vi "Data 2 TypeDescriptor.vi"(8 "error in (no error)":errorcluster, 11 "Data":variant) -> (0 "Error Out":errorcluster, 3 "TypeDescriptor":string)   [LabVIEW 2014, in "CS++Utilities.lvlib"]
uses:
  CS++Utilities.lvlib
  <vilib>/Utility/VariantDataType/VariantType.lvlib
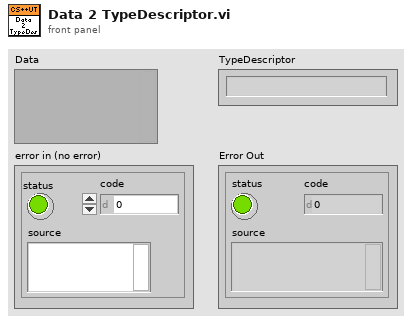
[diagram p1: front panel]
types:
  T1 = typedef "VariantType.lvlib/Type.ctl" = enum8{"Invalid Type", "Void", "I8", "I16", "I32", "I64", "U8", "U16", "U32", "U64", "Single Float", "Double Float", "Extended Float", "Single Complex", "Double Complex", "Extended Complex", "Enum U8", "Enum U16", "Enum U32", "Enum U64", "Single Float With Unit", "Double Float With Unit", "Extended Float With Unit", "Single Complex with Unit", "Double Complex with Unit", "Extended Complex with Unit", "Boolean", "String", "Path", "Picture", "Tag", "Array", "Cluster", "Variant", "LV Variant", "Waveform", "Timestamp", "Digital Waveform", "Digital Data", "ExpressData", "Refnum", "External Data", "VI", "Poly VI", "LabVIEW Class Instance", "Fixed Point"}
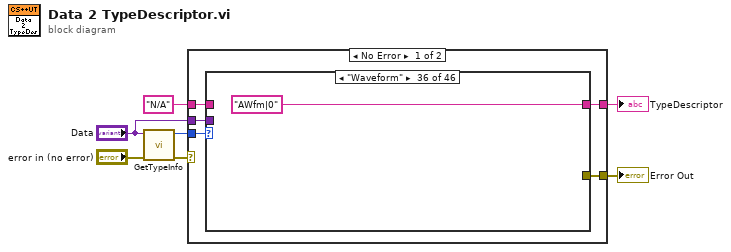
[diagram p0: block diagram]
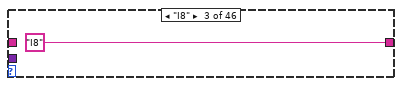
[diagram p4: hidden frame]
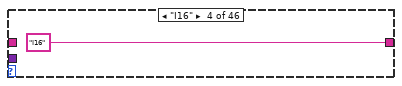
[diagram p5: hidden frame]
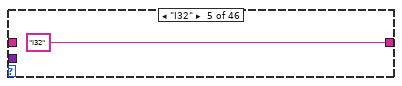
[diagram p6: hidden frame]
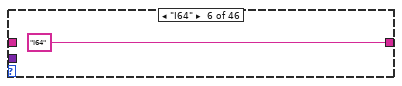
[diagram p7: hidden frame]
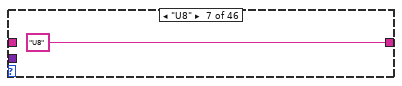
[diagram p8: hidden frame]
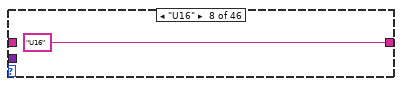
[diagram p9: hidden frame]
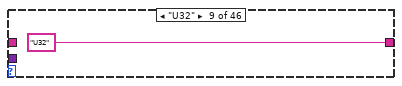
[diagram p10: hidden frame]
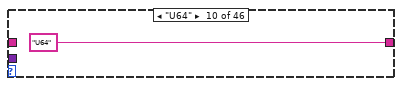
[diagram p11: hidden frame]
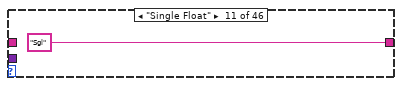
[diagram p12: hidden frame]
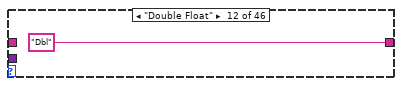
[diagram p13: hidden frame]
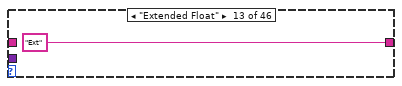
[diagram p14: hidden frame]
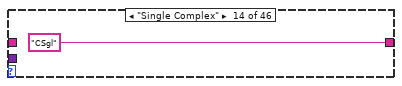
[diagram p15: hidden frame]
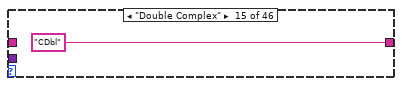
[diagram p16: hidden frame]
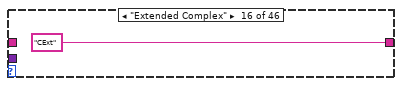
[diagram p17: hidden frame]
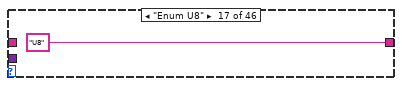
[diagram p18: hidden frame]
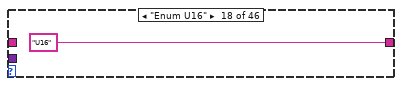
[diagram p19: hidden frame]
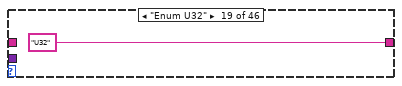
[diagram p20: hidden frame]
diagram:
  n1 = call <vilib>:"GetTypeInfo.vi"("error in (no error)"="error in (no error)", "Variant"="Data") -> ("error out"=w3:errorcluster, "Type Enum"=w7:T1)  [unwired: 5 in, 3 out]
  n2 = case shown="No Error" w3 {
    selector: w3 -> [_ w90]
    tunnel: w7 -> [w12 _]
    tunnel: "Data" -> [w11 _]
    tunnel: [w10 ""] -> w5
    tunnel: [w9 w90] -> w2
    tunnel: "N/A" -> [w8 _]
    frame No Error {
      n3 = case shown="\"Waveform\"" w12 {
        tunnel: w11 -> [_ _ _ _ _ _ _ _ _ _ _ _ _ _ _ _ _ _ _ _ _ _ _ _ _ _ _ _ _ _ _ w47 w68 _ _ _ _ _ _ _ _ _ _ _ _ _]
        tunnel: [w13 w14 "I8" "I16" "I32" "I64" "U8" "U16" "U32" "U64" "Sgl" "Dbl" "Ext" "CSgl" "CDbl" "CExt" "U8" "U16" "U32" "U64" "Sgl" "Dbl" "Ext" "CSgl" "CDbl" "CExt" "Bool" "Str" "Str" w42 w43 w50 w74 w77 w78 "AWfm|0" "T" "DWfm|0" "DD" w83 w84 w85 w86 w87 w88 "FP"] -> w10
        tunnel: [_ _ _ _ _ _ _ _ _ _ _ _ _ _ _ _ _ _ _ _ _ _ _ _ _ _ _ _ _ _ _ w49 w69 _ _ _ _ _ _ _ _ _ _ _ _ _] -> w9
        tunnel: w8 -> [w13 w14 _ _ _ _ _ _ _ _ _ _ _ _ _ _ _ _ _ _ _ _ _ _ _ _ _ _ _ w42 w43 _ _ w77 w78 _ _ _ _ w83 w84 w85 w86 w87 w88 _]
        frame "Invalid Type", Default {
        }
        frame "Void" {
        }
        frame "I8" {
        }
        frame "I16" {
        }
        frame "I32" {
        }
        frame "I64" {
        }
        frame "U8" {
        }
        frame "U16" {
        }
        frame "U32" {
        }
        frame "U64" {
        }
        frame "Single Float" {
        }
        frame "Double Float" {
        }
        frame "Extended Float" {
        }
        frame "Single Complex" {
        }
        frame "Double Complex" {
        }
        frame "Extended Complex" {
        }
        frame "Enum U8" {
        }
        frame "Enum U16" {
        }
        frame "Enum U32" {
        }
        frame "Enum U64" {
        }
        frame "Single Float With Unit" {
        }
        frame "Double Float With Unit" {
        }
        frame "Extended Float With Unit" {
        }
        frame "Single Complex with Unit" {
        }
        frame "Double Complex with Unit" {
        }
        frame "Extended Complex with Unit" {
        }
        frame "Boolean" {
        }
        frame "String" {
        }
        frame "Path" {
        }
        frame "Picture" {
        }
        frame "Tag" {
        }
        frame "Cluster" {
          n4 = call "Cluster to Array of VData__ogtk.vi"("Cluster"=w47) -> ("error out"=w48:errorcluster, "Array of VData"=w46:variant[])  [unwired: 9 in]
          n5 = for "For all cluster elements" {
            tunnel: w46 -> [w61] mode=indexing
            shift-right: [w62] -> w49
            shift-left: w48 -> [w60]
            tunnel: [w59] -> w51 mode=indexing
            i -> [w57]
            n6 = call "Data 2 TypeDescriptor.vi"("error in (no error)"=w60, "Data"=w61) -> ("Error Out"=w62:errorcluster, "TypeDescriptor"=w58:string)  [unwired: 8 in]
            n7 = Equal To 0?(x=w57) -> (x = 0?=w56:bool)
            n8 = Select(t="", s=w56, f=";" ("string")) -> (s? t:f=w55:string)
            n9 = Concatenate Strings(w55, w58) -> (w59:string)
          }
          n10 = Build Array (concatenate)("{", w51, "}") -> (w52:string[])
          n11 = Concatenate Strings(w52) -> (w50:string)
        }
        frame "Array" {
          w64 = ":"
          n12 = call <vilib>:"GetArrayInfo.vi"("Variant"=w68) -> ("error out"=w73:errorcluster, "ArrayElement"=w71:variant)  [unwired: 7 in, 2 out]
          n13 = call "Data 2 TypeDescriptor.vi"("error in (no error)"=w73, "Data"=w71) -> ("Error Out"=w70:errorcluster, "TypeDescriptor"=w72:string)  [unwired: 8 in]
          n14 = call "Array Size(s)__ogtk.vi"("error in (no error)"=w70, "Array"=w68) -> ("error out"=w69:errorcluster, "Size(s)"=w63:u32[])  [unwired: 7 in, 1 out]
          n15 = Number To Decimal String(number=w63) -> (decimal integer string=w66:string[])  [unwired: 1 in]
          n16 = call "String Array 2 String.vi"("Substrings"=w66, "Delimiter (\",\")"=w64) -> ("String"=w65:string)
          n17 = Build Array("[", w72, w64, w65, "]") -> (w75:string[])
          n18 = Concatenate Strings(w75) -> (w74:string)
        }
        frame "Variant" {
        }
        frame "LV Variant" {
        }
        frame "Waveform" {
        }
        frame "Timestamp" {
        }
        frame "Digital Waveform" {
        }
        frame "Digital Data" {
        }
        frame "ExpressData" {
        }
        frame "Refnum" {
        }
        frame "External Data" {
        }
        frame "VI" {
        }
        frame "Poly VI" {
        }
        frame "LabVIEW Class Instance" {
        }
        frame "Fixed Point" {
        }
      }
    }
    frame Error {
    }
  }
  "TypeDescriptor" <- w5
  "Error Out" <- w2
